vi "Generate Waterfall Plot.vi"(9 "number of samples":i64, 10 "Waterfall Time Scale (s)":i32, 11 "power spectrum":cluster{"f0":dbl, "df":dbl, "magnitude":dbl[]}) -> (3 "Waterfall Plot Output":dbl[][](array[numeric]))   [LabVIEW 2014]
doc: "Generates a waterfall plot (spectrogram) from power spectrum data, a given time scale, and the number of samples in the spectrum data."
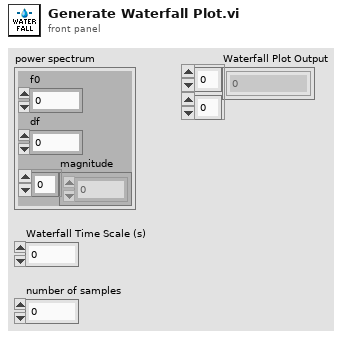
[diagram p1: front panel]
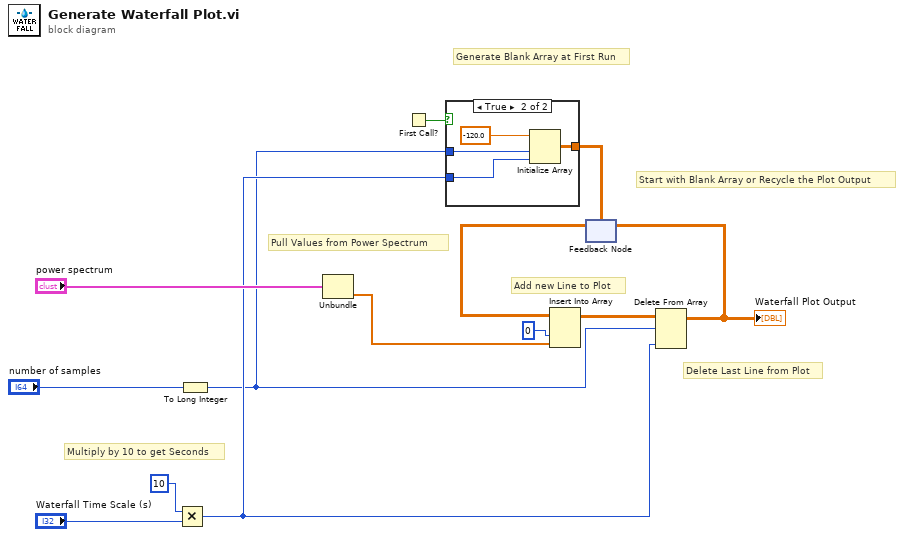
[diagram p0: block diagram]
diagram:
  # "Multiply by 10 to get Seconds"
  # "Start with Blank Array or Recycle the Plot Output"
  # "Delete Last Line from Plot"
  # "Add new Line to Plot"
  # "Pull Values from Power Spectrum"
  # "Generate Blank Array at First Run"
  n1 = Multiply(x=10, y="Waterfall Time Scale (s)") -> (x*y=w12:i32)
  n2 = To Long Integer(number="number of samples") -> (32bit integer=w9:i32)
  n3 = Unbundle("power spectrum") -> ("magnitude"=w1:dbl[])  [unwired: 2 out]
  n4 = First Call?() -> (First Call?: T/F=w4:bool)
  n5 = case shown="True" w4 {
    tunnel: w9 -> [_ w16]
    tunnel: [_ w15] -> w5
    tunnel: w12 -> [_ w14]
    frame False {
    }
    frame True {
      n6 = Initialize Array(-120.0 ("element"), w16, w14) -> (w15:dbl[][])
    }
  }
  n7 = feedback #1(w5) -> (w6:dbl[][])
  n8 = Insert Into Array(array=w6, index (col)=0 ("index (row)"), new element=w1) -> (w2:dbl[][])  [unwired: 1 in]
  n9 = Delete From Array(array=w2, length=w9, index (col)=w12) -> (array with subset deleted=w7:dbl[][])  [unwired: 1 in, 1 out]
  "Waterfall Plot Output" <- w7
  n10 = feedback-in #1(w7) -> ()
